vi "ELVIS III v1.0 Reserve Channel List Core.vi"(7 "Allow multiple opens?":bool, 8 "error in (no error)":errorcluster, 10 "Channel Reservation List":T1, 11 "Owner":string) -> (0 "error out":errorcluster)   [LabVIEW 2021]
uses:
  <vilib>/myRIO/Common/Instrument Driver Framework/ELVIS III v1.0/Resource Manager/typedefs/ELVIS III v1.0 Channel Reservation List.ctl
  <vilib>/myRIO/Common/Instrument Driver Framework/ELVIS III v1.0/Resource Manager/typedefs/ELVIS III v1.0 Channel Reservation Info.ctl
  <vilib>/myRIO/Common/Instrument Driver Framework/ELVIS III v1.0/Resource Manager/typedefs/ELVIS III v1.0 Connector List.ctl
  <vilib>/myRIO/Common/Instrument Driver Framework/ELVIS III v1.0/Resource Manager/vis/ELVIS III v1.0 Build Mutex Name.vi
  <vilib>/myRIO/Common/Instrument Driver Framework/Utilities/vis/IO Manager.vi
  <vilib>/Utility/error.llb/Error Cluster From Error Code.vi
  <vilib>/myRIO/Common/Instrument Driver Framework/Utilities/vis/Configuration Manager.vi
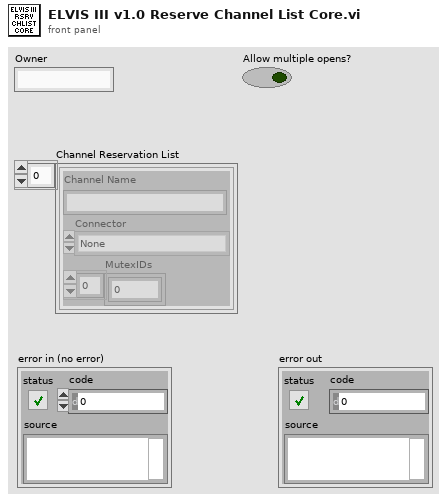
[diagram p1: front panel]
types:
  T1 = typedef "ELVIS III v1.0 Channel Reservation List.ctl" = T2[]
  T2 = typedef "ELVIS III v1.0 Channel Reservation Info.ctl" = cluster{"Channel Name":string, "Connector":T3, "MutexIDs":u32[]}
  T3 = typedef "ELVIS III v1.0 Connector List.ctl" = enum32{"None", "ConnectorA", "ConnectorB"}
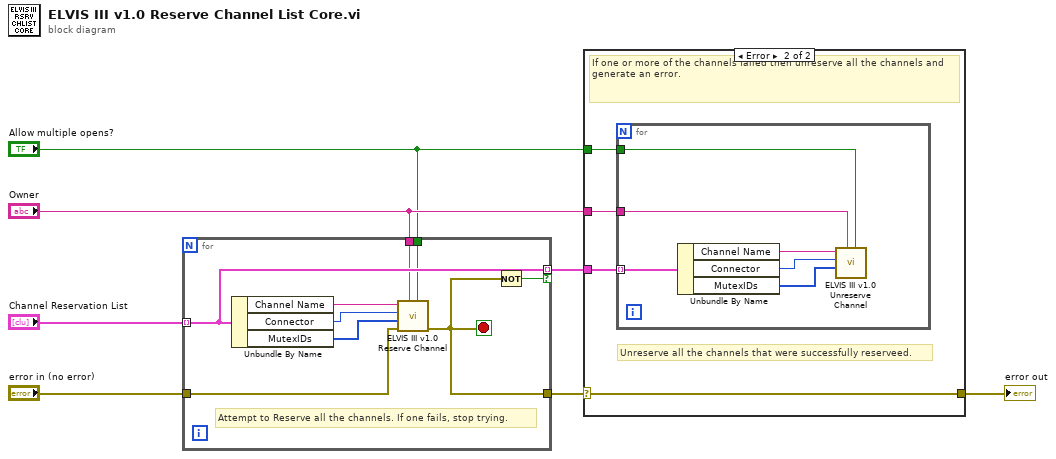
[diagram p0: block diagram]
diagram:
  n1 = for {
    tunnel: "Allow multiple opens?" -> [w14]
    tunnel: [w11] -> w1
    tunnel: "Channel Reservation List" -> [w16] mode=indexing
    tunnel: [w16] -> w3 mode=indexing if=w15
    tunnel: "Owner" -> [w13]
    tunnel: "error in (no error)" -> [w10]
    stop <- w11 stop-if-true
    # "Attempt to Reserve all the channels. If one fails, stop trying."
    n2 = Unbundle By Name(w16) -> ("Channel Name"=w12:string, "Connector"=w9:T3, "MutexIDs"=w8:u32[])
    n3 = call <vilib>:"ELVIS III v1.0 Reserve Channel.vi"("Allow multiple opens?"=w14, "Owner"=w13, "error in (no error)"=w10, "Mutex IDs"=w8, "Connector"=w9, "Channel Name"=w12) -> ("error out"=w11:errorcluster)  [unwired: 5 in]
    n4 = Not(x=w11) -> (.not. x?=w15:bool)
  }
  n5 = case shown="Error" w1 {
    selector: w1 -> [w17 w18]
    tunnel: w3 -> [_ w21]
    tunnel: "Owner" -> [_ w20]
    tunnel: "Allow multiple opens?" -> [_ w19]
    tunnel: [w17 w18] -> w5
    frame No Error {
      # "If all channels were successfully reserved then there is nothing to do."
    }
    frame Error {
      # "Unreserve all the channels that were successfully reserveed."
      # "If one or more of the channels failed then unreserve all the channels and generate an error."
      n6 = for {
        tunnel: w21 -> [w23] mode=indexing
        tunnel: w20 -> [w26]
        tunnel: w19 -> [w27]
        n7 = Unbundle By Name(w23) -> ("Channel Name"=w25:string, "Connector"=w24:T3, "MutexIDs"=w22:u32[])
        n8 = call <vilib>:"ELVIS III v1.0 Unreserve Channel.vi"("Allow multiple opens?"=w27, "Owner"=w26, "Mutex IDS"=w22, "Connector"=w24, "Channel Name"=w25) -> ()  [unwired: 6 in, 1 out]
      }
    }
  }
  "error out" <- w5
